vi "Asylum_Driver_PostObjectInitialize.vi"(4 "Abort Notifier":refnum<notifier>, 8 "error in (no error)":errorcluster, 9 "Offsets":cluster{"X":dbl, "Y":dbl}, 10 "Pattern Data":T2, 11 "Application In":refnum<k7>) -> (0 "error out":errorcluster, 3 "Application Out":refnum<k7>)   [LabVIEW 2019]
uses:
  <userlib>/LevyLab/Relay Box/Typedefs/Resistor--enum.ctl
  44659c71-bd9a-4326-9702-5dd3a5981512.vi
  44659c71-bd9a-4326-9702-5dd3a5981512.vi/34e17190-a4ef-4b57-a1ea-52a2bfeb3336.vi
  <vilib>/Utility/Debug Log/Display.vi
  <userlib>/LevyLab/Relay Box/Relay-Box.lvclass
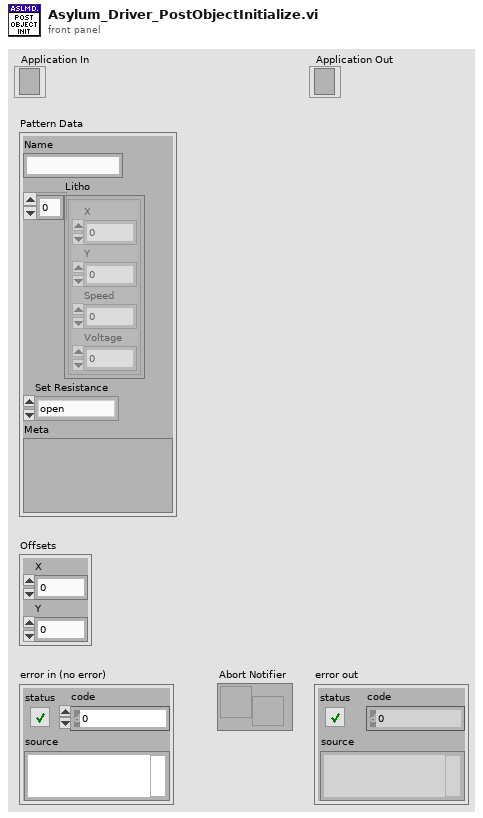
[diagram p1: front panel]
types:
  T1 = typedef "Relay-Box.lvclass/Resistor--enum.ctl" = enum16{"open", "discharge tip", "0 ohms", "100k ohm", "10M ohm", "1G ohm"}
  T2 = cluster{"Name":string, "Litho":cluster{"X":dbl, "Y":dbl, "Speed":dbl, "Voltage":dbl}[], "Set Resistance":T1, "Meta":variant}
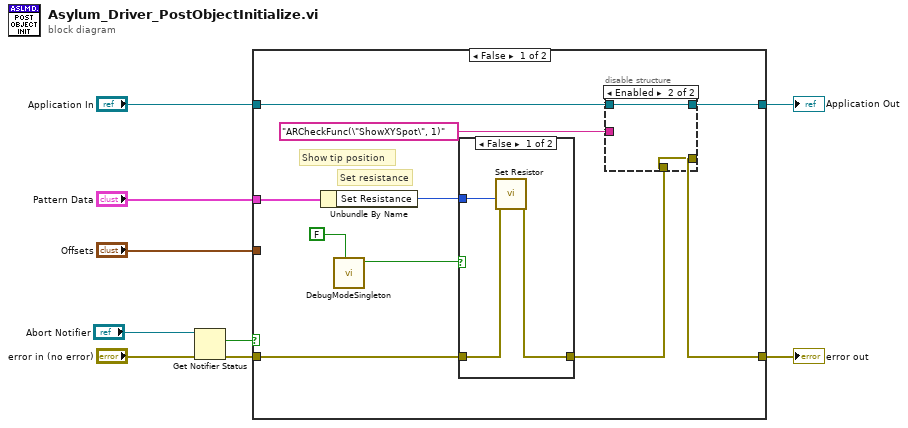
[diagram p0: block diagram]
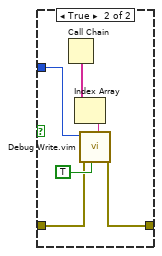
[diagram p2: hidden frame]
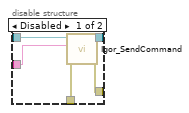
[diagram p3: hidden frame]
diagram:
  n1 = Get Notifier Status(notifier="Abort Notifier", error in (no error)="error in (no error)") -> (current notification=w4:bool, error out=w6:errorcluster)  [unwired: 3 out]
  n2 = case shown="False" w4 {
    tunnel: [w15 w37] -> w9
    tunnel: "Pattern Data" -> [w18 _]
    tunnel: w6 -> [w12 w37]
    tunnel: [w16 w36] -> w3
    tunnel: "Application In" -> [w17 w36]
    tunnel: "Offsets" -> [_ _]
    frame False {
      # "Show tip position"
      # "Set resistance"
      n3 = Unbundle By Name(w18) -> ("Set Resistance"=w19:T1)
      n4 = call <userlib>:"DebugModeSingleton.vi"("Write?"=FALSE) -> ("Debug Mode?"=w11:bool)  [unwired: 10 in]
      n5 = case shown="False" w11 {
        tunnel: w19 -> [w22 w28]
        tunnel: [w21 w24] -> w13
        tunnel: w12 -> [w20 w23]
        frame False {
          n6 = call <userlib>:"Set Resistor.vi"("error in"=w20, "Set Resistance"=w22) -> ("error out"=w21:errorcluster)  [unwired: 9 in]
        }
        frame True {
          n7 = Call Chain() -> (call chain=w27:string[])
          n8 = Index Array(array=w27) -> (element=w26:string)  [unwired: 1 in]
          n9 = call "Debug Write.vim"("include timestamp? (F)"=TRUE, "prefix (\"\")"=w26, "error in (no error)"=w23, "value"=w28) -> ("error out"=w24:errorcluster)  [unwired: 7 in]
        }
      }
      n10 = disable-structure shown="Enabled" {
        disable-tunnel: w17 -> [w33 w35]
        disable-tunnel: [w32 w35] -> w16
        disable-tunnel: w13 -> [w31 w34]
        disable-tunnel: [w30 w34] -> w15
        disable-tunnel: "ARCheckFunc(\"ShowXYSpot\", 1)" ("parameterName") -> [w29 _]
        frame Disabled {
          n11 = call <userlib>:"Igor_SendCommand.vi"("error in (no error)"=w31, "command"=w29, "Application In"=w33) -> ("error out"=w30:errorcluster, "Application Out"=w32:refnum<k7>)  [unwired: 5 in, 2 out]
        }
        frame Enabled {
        }
      }
    }
    frame True {
      # "Abort has been called. Don't do anything new here"
    }
  }
  "error out" <- w9
  "Application Out" <- w3
